vi "Response Class Type.vi"(11 "Type":string) -> (3 "Class":refnum<class "Response.lvclass">)   [LabVIEW 2022 SP3, in "obs-websocket-lv.lvlib"]
uses:
  obs-websocket-lv.lvlib
  Response/Response.lvclass
  RGetSourceScreenshot/RGetSourceScreenshot.lvclass
  C:/dev/illuminatedg/obs-websocket-lv/obs-websocket-lv/Response/Response.lvclass
  RGetSceneList/RGetSceneList.lvclass
  RGetCurrentProgramScene/RGetCurrentProgramScene.lvclass
  RGetStreamStatus/RGetStreamStatus.lvclass
  RJSONDebug/RJSONDebug.lvclass
  RGetInputList/RGetInputList.lvclass
  RGetInputVolume/RGetInputVolume.lvclass
  REmptyResponse/REmptyResponse.lvclass
  RGetSceneItemID/RGetSceneItemID.lvclass
  RGetSceneItemEnabled/RGetSceneItemEnabled.lvclass
  RGetInputMute/RGetInputMute.lvclass
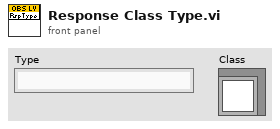
[diagram p1: front panel]
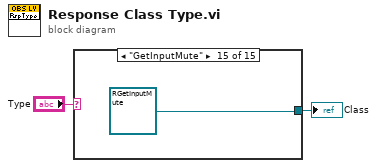
[diagram p0: block diagram]
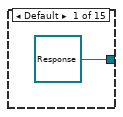
[diagram p2: hidden frame]
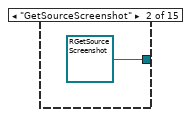
[diagram p3: hidden frame]
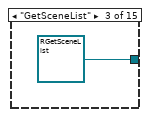
[diagram p4: hidden frame]
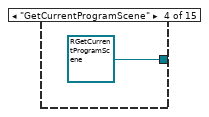
[diagram p5: hidden frame]
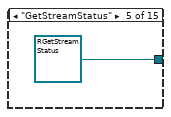
[diagram p6: hidden frame]
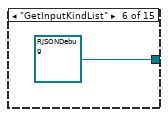
[diagram p7: hidden frame]
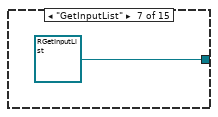
[diagram p8: hidden frame]
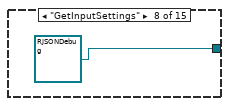
[diagram p9: hidden frame]
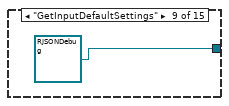
[diagram p10: hidden frame]
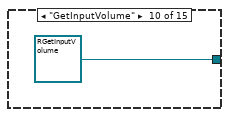
[diagram p11: hidden frame]
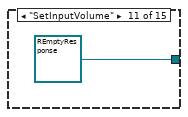
[diagram p12: hidden frame]
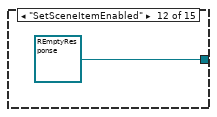
[diagram p13: hidden frame]
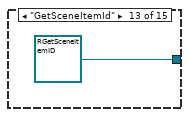
[diagram p14: hidden frame]
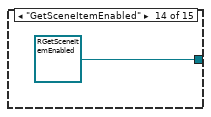
[diagram p15: hidden frame]
diagram:
  n1 = case shown="\"GetInputMute\"" "Type" {
    tunnel: [refnum<class "Response.lvclass"> refnum ("obs-websocket-lv.lvlib:Response.lvclass") refnum<class "RGetSourceScreenshot.lvclass"> refnum ("obs-websocket-lv.lvlib:RGetSourceScreenshot.lvclass") refnum<class "RGetSceneList.lvclass"> refnum ("obs-websocket-lv.lvlib:RGetSceneList.lvclass") refnum<class "RGetCurrentProgramScene.lvclass"> refnum ("obs-websocket-lv.lvlib:RGetCurrentProgramScene.lvclass") refnum<class "RGetStreamStatus.lvclass"> refnum ("obs-websocket-lv.lvlib:RGetStreamStatus.lvclass") refnum<class "RJSONDebug.lvclass"> refnum ("obs-websocket-lv.lvlib:RJSONDebug.lvclass") refnum<class "RGetInputList.lvclass"> refnum ("obs-websocket-lv.lvlib:RGetInputList.lvclass") refnum<class "RJSONDebug.lvclass"> refnum ("obs-websocket-lv.lvlib:RJSONDebug.lvclass") refnum<class "RJSONDebug.lvclass"> refnum ("obs-websocket-lv.lvlib:RJSONDebug.lvclass") refnum<class "RGetInputVolume.lvclass"> refnum ("obs-websocket-lv.lvlib:RGetInputVolume.lvclass") refnum<class "REmptyResponse.lvclass"> refnum ("obs-websocket-lv.lvlib:REmptyResponse.lvclass") refnum<class "REmptyResponse.lvclass"> refnum ("obs-websocket-lv.lvlib:REmptyResponse.lvclass") refnum<class "RGetSceneItemID.lvclass"> refnum ("obs-websocket-lv.lvlib:RGetSceneItemID.lvclass") refnum<class "RGetSceneItemEnabled.lvclass"> refnum ("obs-websocket-lv.lvlib:RGetSceneItemEnabled.lvclass") refnum<class "RGetInputMute.lvclass"> refnum ("obs-websocket-lv.lvlib:RGetInputMute.lvclass")] -> w1
    frame Default {
    }
    frame "GetSourceScreenshot" {
    }
    frame "GetSceneList" {
    }
    frame "GetCurrentProgramScene" {
    }
    frame "GetStreamStatus" {
    }
    frame "GetInputKindList" {
    }
    frame "GetInputList" {
    }
    frame "GetInputSettings" {
    }
    frame "GetInputDefaultSettings" {
    }
    frame "GetInputVolume" {
    }
    frame "SetInputVolume" {
    }
    frame "SetSceneItemEnabled" {
    }
    frame "GetSceneItemId" {
    }
    frame "GetSceneItemEnabled" {
    }
    frame "GetInputMute" {
    }
  }
  "Class" <- w1
